vi "Configuration - Determine Device Type String.vi"(10 "Device Type In":T1) -> (2 "Type String Out":string)   [LabVIEW 2017, in "Communications Library.lvlib"]
uses:
  Communications Library.lvlib
  Typedefs/DTACQ Device Type--Enum.ctl
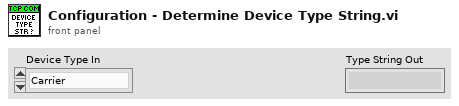
[diagram p1: front panel]
types:
  T1 = typedef "Communications Library.lvlib/DTACQ Device Type--Enum.ctl" = enum16{"Carrier", "Analog In Module", "Analog Out Module", "Generic Module"}
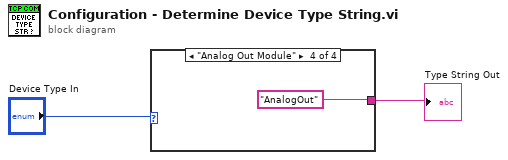
[diagram p0: block diagram]
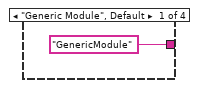
[diagram p2: hidden frame]
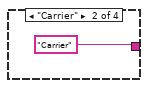
[diagram p3: hidden frame]
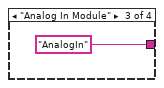
[diagram p4: hidden frame]
diagram:
  n1 = case shown="\"Analog Out Module\"" "Device Type In" {
    tunnel: ["GenericModule" "Carrier" "AnalogIn" "AnalogOut"] -> w1
    frame "Generic Module", Default {
    }
    frame "Carrier" {
    }
    frame "Analog In Module" {
    }
    frame "Analog Out Module" {
    }
  }
  "Type String Out" <- w1
